vi "Destructor.vi"(8 "error in":errorcluster, 11 "SequenceRunReference in":refnum<class "SequenceRunReference.lvclass">) -> (0 "error out":errorcluster)   [LabVIEW 2021, in "ProligentXMLGenerator.lvlib" / "SequenceRunReference.lvclass"]
uses:
  SequenceRunReference.lvclass
  SequenceRunReference.lvclass/SequenceRunReference.ctl
  Model/CustomData/CustomData.lvclass
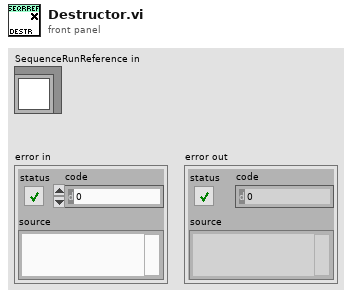
[diagram p1: front panel]
types:
  T1 = typedef "ProligentXMLGenerator.lvlib/SequenceRunReference.lvclass/Data.ctl" = cluster{"Name":string, "CustomData":refnum<class "CustomData.lvclass">, "Id":refnum<class "Guid.lvclass">}
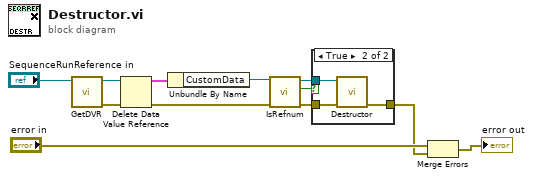
[diagram p0: block diagram]
diagram:
  n1 = call "GetDVR.vi"("SequenceRunReference in"="SequenceRunReference in") -> ("error out"=w9:errorcluster, "DVRReference"=w10:refnum<data-value>)  [unwired: 9 in]
  n2 = Delete Data Value Reference(data value reference=w10, error in=w9) -> (data value=w8:T1, error out=w1:errorcluster)
  n3 = Unbundle By Name(w8) -> ("CustomData"=w4:refnum<class "CustomData.lvclass">)
  n4 = call "IsRefnum.vi"("error in"=w1, "CustomDataType in"=w4) -> ("error out"=w6:errorcluster, "IsRefnum"=w5:bool, "CustomDataType out"=w2:refnum<class "CustomData.lvclass">)  [unwired: 7 in]
  n5 = case shown="True" w5 {
    tunnel: w6 -> [w13 w16]
    tunnel: [w13 w15] -> w3
    tunnel: w2 -> [_ w14]
    frame False {
    }
    frame True {
      n6 = call "Destructor.vi"("error in"=w16, "CustomDataType"=w14) -> ("error out"=w15:errorcluster)  [unwired: 9 in]
    }
  }
  n7 = Merge Errors("error in", w3) -> (→"error out":errorcluster)
